vi "Scrub.vi"(8 "error in":errorcluster, 10 "Input String":string, 11 "Multi Scrubber in":refnum<class "Multi Scrubber.lvclass">) -> (0 "error out":errorcluster, 2 "Scrubbed String":string, 3 "Multi Scrubber out":refnum<class "Multi Scrubber.lvclass">)   [LabVIEW 2020, in "Approval Tests.lvlib" / "Multi Scrubber.lvclass"]
uses:
  Multi Scrubber.lvclass
  Multi Scrubber.lvclass/Multi Scrubber.ctl
  Scrubber/Scrubber.lvclass
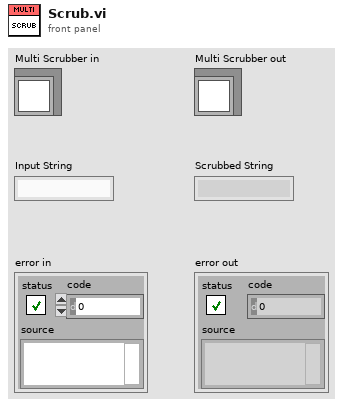
[diagram p1: front panel]
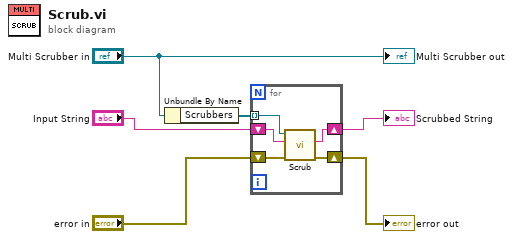
[diagram p0: block diagram]
diagram:
  n1 = Unbundle By Name("Multi Scrubber in") -> ("Scrubbers"=w3:refnum<class "Scrubber.lvclass">[])
  n2 = for {
    tunnel: w3 -> [w9] mode=indexing
    shift-right: [w7] -> w1
    shift-left: "Input String" -> [w8]
    shift-right: [w10] -> w5
    shift-left: "error in" -> [w11]
    n3 = call-dynamic "Scrub.vi"("error in"=w11, "Input String"=w8, "Scrubber in"=w9) -> ("error out"=w10:errorcluster, "Scrubbed String"=w7:string)  [unwired: 6 in, 1 out]
  }
  "error out" <- w5
  "Scrubbed String" <- w1
  "Multi Scrubber out" <- "Multi Scrubber in"
